vi "Update Tiles Info.vi"(8 "error in (no error)":errorcluster, 11 "Sensor Model in":refnum<class "Sensor Model.lvclass">) -> (0 "error out":errorcluster, 3 "Sensor Model out":refnum<class "Sensor Model.lvclass">)   [LabVIEW 2013, in "Sensor Model.lvlib" / "Sensor Model.lvclass"]
uses:
  Sensor Model.lvclass
  Sensor Model.lvclass/Sensor Model.ctl
  <vilib>/ActorFrameworkMVC/View Observer/View Registry/View Registry.lvclass/View Registry.ctl
  Sensor Model Messages/Abstract Sensor Tiles Info Msg/Abstract Sensor Tiles Info Msg.lvclass
  <vilib>/ActorFrameworkMVC/View Observer/Data Message/Data Message.lvclass
  <vilib>/ActorFrameworkMVC/View Observer/View Registry/View Registry.lvclass
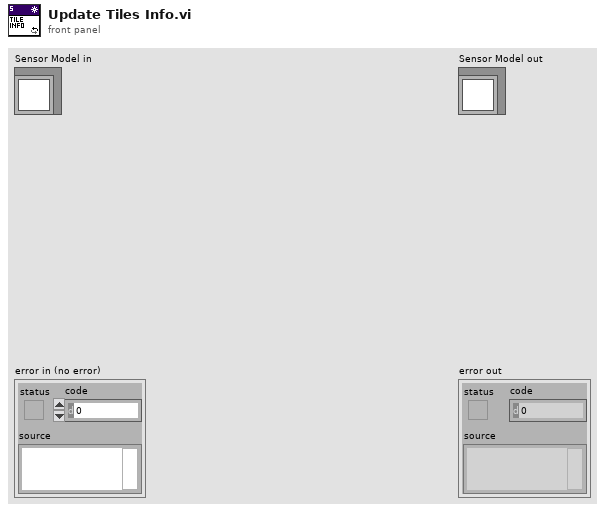
[diagram p1: front panel]
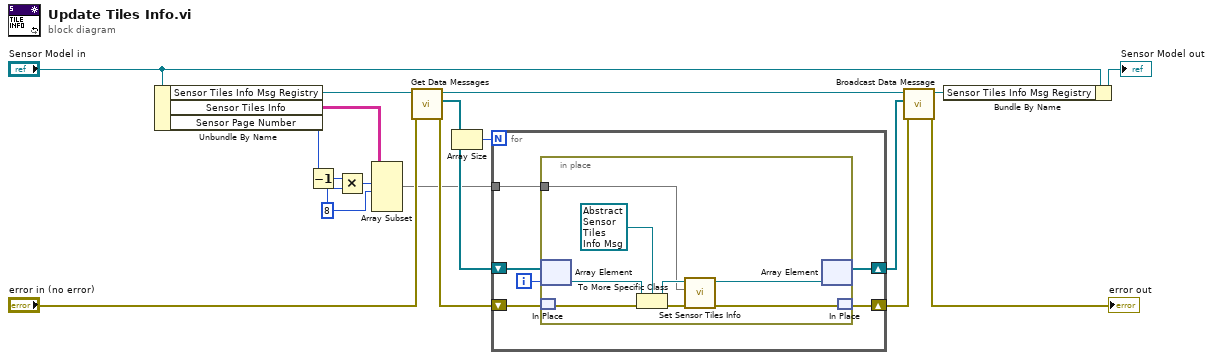
[diagram p0: block diagram]
diagram:
  w3 = 8 ("length")
  n1 = Unbundle By Name("Sensor Model in") -> ("Sensor Tiles Info Msg Registry"=w18:refnum<class "View Registry.lvclass">, "Sensor Tiles Info"=w2:string[][], "Sensor Page Number"=w4:i32)
  n2 = Decrement(x=w4) -> (x-1=w5:i32)
  n3 = Multiply(x=w5, y=w3) -> (x*y=w6:i32)
  n4 = Array Subset(array=w2, index (row)=w6, length (row)=w3) -> (w1:string[][])  [unwired: 2 in]
  n5 = call <vilib>:"Get Data Messages.vi"("error in (no error)"="error in (no error)", "View Registry in"=w18) -> ("error out"=w14:errorcluster, "Data Messages"=w15:refnum<class "Data Message.lvclass">[], "View Registry out"=w17:refnum<class "View Registry.lvclass">)  [unwired: 7 in]
  n6 = Array Size(array=w15) -> (size(s)=w16:i32)
  n7 = for {
    N: w16 -> [_]
    shift-right: [w23] -> w13
    shift-left: w15 -> [w24]
    shift-right: [w20] -> w12
    shift-left: w14 -> [w22]
    tunnel: w1 -> [w21]
    i -> [w19]
    n8 = in-place {
      in-place-border: w21 -> [w25]
      n9 = in-place-array #1(w24, w19) -> (w30:refnum<class "Data Message.lvclass">)
      n10 = in-place-match #2(w22) -> (w32:errorcluster)
      n11 = To More Specific Class(target class=refnum<class "Abstract Sensor Tiles Info Msg.lvclass"> refnum ("Sensor Model.lvlib:Abstract Sensor Tiles Info Msg.lvclass"), reference=w30, error in=w32) -> (specific class reference=w26:refnum<class "Abstract Sensor Tiles Info Msg.lvclass">, error out=w29:errorcluster)
      n12 = call "Set Sensor Tiles Info.vi"("error in (no error)"=w29, "Sensor Tiles Info"=w25, "Abstract Sensor Tiles Info Msg in"=w26) -> ("error out"=w28:errorcluster, "Abstract Sensor Tiles Info Msg out"=w27:refnum<class "Abstract Sensor Tiles Info Msg.lvclass">)  [unwired: 7 in]
      n13 = in-place-array #1(w27) -> (w23:refnum<class "Data Message.lvclass">[])  [unwired: 1 out]
      n14 = in-place-match #2(w28) -> (w20:errorcluster)
    }
  }
  n15 = call <vilib>:"Broadcast Data Message.vi"("error in (no error)"=w12, "Data Messages"=w13, "View Registry in"=w17) -> ("error out"=→"error out":errorcluster, "View Registry out"=w11:refnum<class "View Registry.lvclass">)  [unwired: 7 in]
  n16 = Bundle By Name(cluster="Sensor Model in", "Sensor Tiles Info Msg Registry"=w11) -> (→"Sensor Model out":refnum<class "Sensor Model.lvclass">)
